vi "UDT_lowLevelControllerModule_enableMotors.vi"() -> (3 "Unit Test Framework Results":T1)   [LabVIEW 2017]
doc: "Use this template to create a user-defined test VI. Define your test requirements and wire the results to the <b>Result (Test)</b> control. Do not modify the <b>Unit Test Framework Results</b> indicator."
uses:
  <vilib>/utf/common/utf_test_result_troll.ctl
  <vilib>/utf/common/utf_test_result.ctl
  <vilib>/utf/common/utf_test_result_failure.ctl
  <vilib>/utf/common/utf_test_comparison_operators.ctl
  <vilib>/utf/common/utf_vi_tag.ctl
  RT/ErrorMonitor/Queue/TypeDefs/queueFGVState.ctl
  <vilib>/Control Software Solutions Ltd/UTF Helper/SubVIs/UTF Boolean Equals.vi
  RT/ErrorMonitor/ErrorMonitor.lvlib
  <vilib>/Control Software Solutions Ltd/UTF Helper/Unit Test Helper.lvlib
  RT/LowLevelController/lowLevelController.lvlib
  <vilib>/utf/NI_UnitTestFramework.lvlib
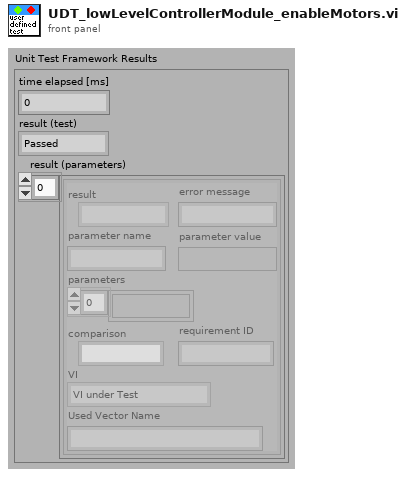
[diagram p1: front panel]
types:
  T1 = typedef "NI_UnitTestFramework.lvlib/utf_test_result_troll.ctl" = cluster{"time elapsed [ms]":u32, "result (test)":T2, "result (parameters)":T3[]}
  T2 = typedef "NI_UnitTestFramework.lvlib/utf_test_result.ctl" = enum16{"Passed", "Failed", "Error", "Skipped", "Not Processed"}
  T3 = typedef "NI_UnitTestFramework.lvlib/utf_test_result_failure.ctl" = cluster{"result":T2, "error message":string, "parameter name":string, "parameter value":variant, "parameters":variant[], "comparison":T4, "requirement ID":string, "VI":T5, "Used Vector Name":string}
  T4 = typedef "NI_UnitTestFramework.lvlib/utf_test_comparison_operators.ctl" = enum16{"=", "!=", ">", ">=", "<", "<=", "range", "symmetric tolerance", "asymmetric tolerance", "string contains", "string not contain", "array size", "string length", "array range", "by element", "array range (limit array)", "user-defined", "array contains", "array not contain", "vector length", "= (elm)", "!= (elm)", "= (case insensitive)", "!= (case insensitive)"}
  T5 = typedef "NI_UnitTestFramework.lvlib/utf_vi_tag.ctl" = enum16{"Setup VI", "VI under Test", "Teardown VI"}
  T6 = typedef "ErrorMonitor.lvlib/queueFGVState.ctl" = enum16{"obtain", "enqueue low priority", "enqueue high priority", "dequeue", "release"}
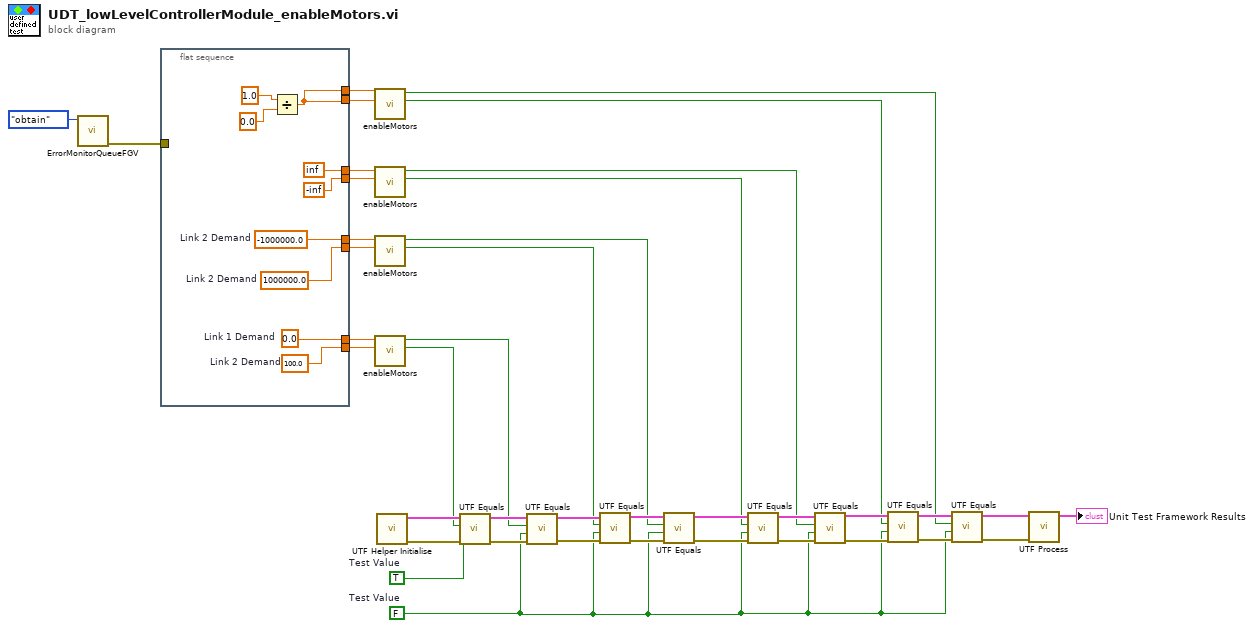
[diagram p0: block diagram]
diagram:
  w19 = FALSE  # Test Value
  w29 = TRUE  # Test Value
  n1 = call "ErrorMonitorQueueFGV.vi"("Enum"=queueFGVState."obtain") -> ("error out"=w38:errorcluster)  [unwired: 9 in, 1 out]
  n2 = flat-sequence {
    tunnel: [w48] -> w6
    tunnel: [w47] -> w5
    tunnel: [w46] -> w7
    tunnel: [w45] -> w8
    tunnel: [inf] -> w12
    tunnel: [-inf] -> w11
    tunnel: [w40] -> w16
    tunnel: w38 -> [_]
    tunnel: [w40] -> w15
    frame #0 {
      w45 = -1000000.0  # Link 2 Demand
      w46 = 1000000.0  # Link 2 Demand
      w47 = 100.0  # Link 2 Demand
      w48 = 0.0  # Link 1 Demand
      n3 = Divide(x=1.0, y=0.0) -> (x/y=w40:dbl)
    }
  }
  n4 = call "enableMotors.vi"("Link 2 Demand"=w15, "Link 1 Demand"=w16) -> ("Enable motor 2"=w13:bool, "Enable motor 1"=w14:bool)  [unwired: 7 in, 1 out]
  n5 = call "enableMotors.vi"("Link 2 Demand"=w11, "Link 1 Demand"=w12) -> ("Enable motor 2"=w9:bool, "Enable motor 1"=w10:bool)  [unwired: 7 in, 1 out]
  n6 = call "enableMotors.vi"("Link 2 Demand"=w7, "Link 1 Demand"=w8) -> ("Enable motor 2"=w3:bool, "Enable motor 1"=w4:bool)  [unwired: 7 in, 1 out]
  n7 = call "enableMotors.vi"("Link 2 Demand"=w5, "Link 1 Demand"=w6) -> ("Enable motor 2"=w1:bool, "Enable motor 1"=w2:bool)  [unwired: 7 in, 1 out]
  n8 = call <vilib>:"UTF Helper Initialise.vi"() -> ("error out"=w30:errorcluster, "results array"=w37:T3[])  [unwired: 10 in]
  n9 = call-poly <vilib>:"UTF Equals.vi"("error in (no error)"=w30, "Test Value"=w29, "Input"=w1, "Input Results"=w37) -> ("error out"=w31:errorcluster, "Output Results"=w36:T3[])  [unwired: 6 in]
  n10 = call-poly <vilib>:"UTF Equals.vi"("error in (no error)"=w31, "Test Value"=w19, "Input"=w2, "Input Results"=w36) -> ("error out"=w32:errorcluster, "Output Results"=w35:T3[])  [unwired: 6 in]
  n11 = call-poly <vilib>:"UTF Equals.vi"("error in (no error)"=w32, "Test Value"=w19, "Input"=w3, "Input Results"=w35) -> ("error out"=w33:errorcluster, "Output Results"=w34:T3[])  [unwired: 6 in]
  n12 = call-poly <vilib>:"UTF Equals.vi"("error in (no error)"=w33, "Test Value"=w19, "Input"=w4, "Input Results"=w34) -> ("error out"=w28:errorcluster, "Output Results"=w20:T3[])  [unwired: 6 in]
  n13 = call-poly <vilib>:"UTF Equals.vi"("error in (no error)"=w28, "Test Value"=w19, "Input"=w9, "Input Results"=w20) -> ("error out"=w27:errorcluster, "Output Results"=w21:T3[])  [unwired: 6 in]
  n14 = call-poly <vilib>:"UTF Equals.vi"("error in (no error)"=w27, "Test Value"=w19, "Input"=w10, "Input Results"=w21) -> ("error out"=w26:errorcluster, "Output Results"=w22:T3[])  [unwired: 6 in]
  n15 = call-poly <vilib>:"UTF Equals.vi"("error in (no error)"=w26, "Test Value"=w19, "Input"=w13, "Input Results"=w22) -> ("error out"=w25:errorcluster, "Output Results"=w23:T3[])  [unwired: 6 in]
  n16 = call-poly <vilib>:"UTF Equals.vi"("error in (no error)"=w25, "Test Value"=w19, "Input"=w14, "Input Results"=w23) -> ("error out"=w18:errorcluster, "Output Results"=w24:T3[])  [unwired: 6 in]
  n17 = call <vilib>:"UTF Process.vi"("error in (no error)"=w18, "results array"=w24) -> ("Unit Test Framework Results"=→"Unit Test Framework Results":T1)  [unwired: 9 in]
